vi "resetNumberOfSavedImages.vi"(8 "error in (no error)":errorcluster, 11 "AndorIKonAcquisitor in":refnum<class "AndorIKonAcquisitor.lvclass">) -> (0 "error out":errorcluster, 3 "AndorIKonAcquisitor out":refnum<class "AndorIKonAcquisitor.lvclass">)   [LabVIEW 2009, in "Hardware.lvlib" / "Channels.lvlib" / "AndorIKonAcquisitor.lvclass"]
uses:
  AndorIKonAcquisitor.lvclass
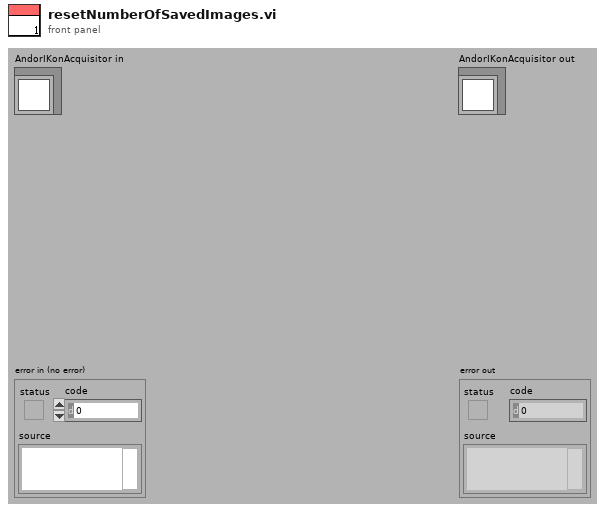
[diagram p1: front panel]
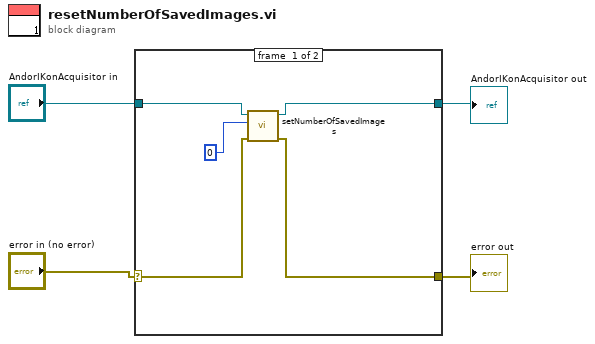
[diagram p0: block diagram]
diagram:
  n1 = case shown="No Error" "error in (no error)" {
    selector: "error in (no error)" -> [w8 w11]
    tunnel: [w5 w11] -> w3
    tunnel: "AndorIKonAcquisitor in" -> [w9 w10]
    tunnel: [w6 w10] -> w1
    frame #0 {
      n2 = call "setNumberOfSavedImages.vi"("error in (no error)"=w8, "NumberOfSavedImages"=0, "AndorIKonAcquisitor.lvclass in"=w9) -> ("error out"=w5:errorcluster, "AndorIKonAcquisitor.lvclass out"=w6:refnum<class "AndorIKonAcquisitor.lvclass">)  [unwired: 7 in]
    }
    frame #1 {
    }
  }
  "error out" <- w3
  "AndorIKonAcquisitor out" <- w1
